vi "GetUniqueFilename.vi"(9 "Enum":T1(ring), 10 "Input path":path) -> (2 "Output path":path)   [LabVIEW 2017]
doc: "Create a unique filename, or return given filename if it does not already exist."
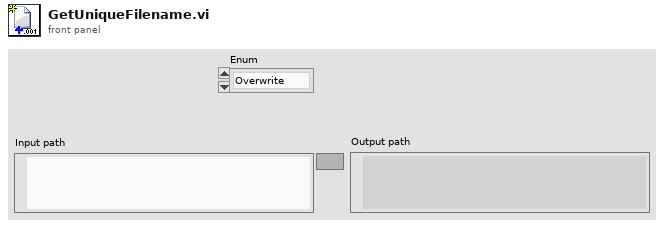
[diagram p1: front panel]
types:
  T1 = enum16{"Overwrite", "Append number", "Append date & time"}
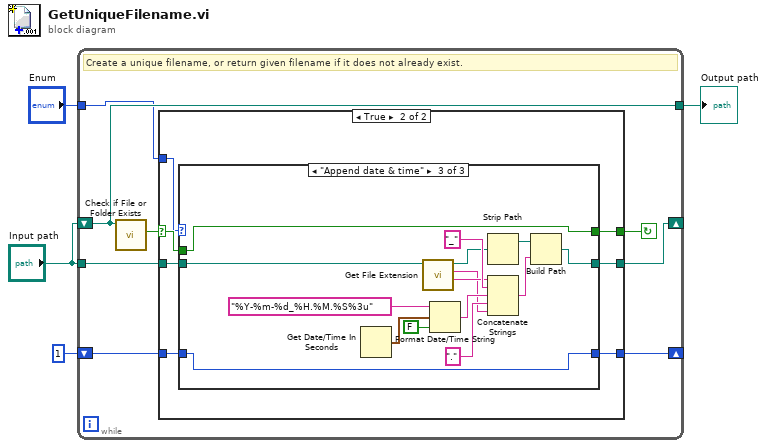
[diagram p0: block diagram]
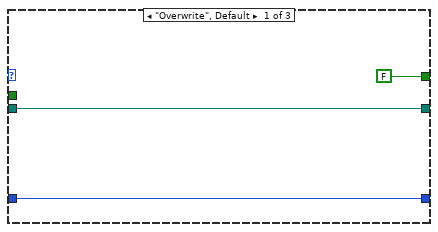
[diagram p3: hidden frame]
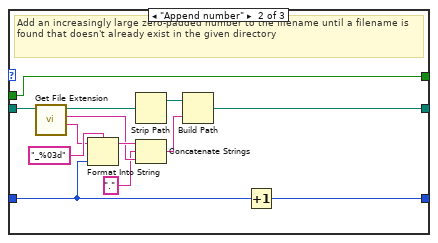
[diagram p4: hidden frame]
diagram:
  n1 = while {
    shift-right: [w10] -> _
    shift-left: "Input path" -> [w12]
    tunnel: [w12] -> w4
    shift-right: [w8] -> _
    shift-left: 1 -> [w9]
    tunnel: "Input path" -> [w7]
    tunnel: "Enum" -> [w5]
    stop <- w11 continue-if-true
    # "Create a unique filename, or return given filename if it does not already exist."
    n2 = call <vilib>:"Check if File or Folder Exists.vi"("path"=w12) -> ("file or folder exists?"=w6:bool)  [unwired: 8 in, 2 out]
    n3 = case shown="True" w6 {
      selector: w6 -> [w14 w17]
      tunnel: [w14 w22] -> w11
      tunnel: [w15 w21] -> w10
      tunnel: w9 -> [w13 w20]
      tunnel: [w13 w19] -> w8
      tunnel: w7 -> [w15 w18]
      tunnel: w5 -> [_ w16]
      frame False {
      }
      frame True {
        n4 = case shown="\"Append date & time\"" w16 {
          tunnel: w18 -> [w24 w36 w49]
          tunnel: w17 -> [_ w38 w53]
          tunnel: [FALSE w38 w53] -> w22
          tunnel: [w24 w33 w46] -> w21
          tunnel: w20 -> [w23 w32 w43]
          tunnel: [w23 w31 w43] -> w19
          frame "Overwrite", Default {
          }
          frame "Append number" {
            # "Add an increasingly large zero-padded number to the filename until a filename is found that doesn't already exist in the given directory"
            n5 = call <vilib>:"Get File Extension.vi"("file"=w36) -> ("filename without extension"=w29:string, "lowercase file extension"=w27:string, "dup file"=w30:path)  [unwired: 6 in, 2 out]
            n6 = Format Into String(format string="_%03d", initial string=w29, w32) -> (resulting string=w34:string)  [unwired: 1 in, 1 out]
            n7 = Strip Path(path=w30) -> (stripped path=w37:path)  [unwired: 1 out]
            n8 = Concatenate Strings(w34, "." ("string"), w27) -> (w28:string)
            n9 = Build Path(base path=w37, name or relative path=w28) -> (appended path=w33:path)
            n10 = Increment(x=w32) -> (x+1=w31:i32)
          }
          frame "Append date & time" {
            n11 = Get Date/Time In Seconds() -> (seconds since 1Jan1904=w52:timestamp)
            n12 = call <vilib>:"Get File Extension.vi"("file"=w49) -> ("filename without extension"=w41:string, "lowercase file extension"=w39:string, "dup file"=w42:path)  [unwired: 6 in, 2 out]
            n13 = Format Date/Time String(time format string (%c)="%Y-%m-%d_%H.%M.%S%3u", seconds (now)=w52, UTC format=FALSE) -> (date/time string=w45:string)
            n14 = Strip Path(path=w42) -> (stripped path=w48:path)  [unwired: 1 out]
            n15 = Concatenate Strings(w41, "_" ("string"), w45, "." ("string"), w39) -> (w47:string)
            n16 = Build Path(base path=w48, name or relative path=w47) -> (appended path=w46:path)
          }
        }
      }
    }
  }
  "Output path" <- w4
